vi "Create Group.vi"(4 "Channel Resources (Unset)":string[](array[string]), 5 "Raw Values (F)":bool, 6 "Channel Names":string[](array[string]), 7 "Group Type":refnum<class "Group.lvclass">, 8 "error in (no error)":errorcluster, 9 "Multicast Config (None)":T1, 10 "Group Info":T2, 11 "VolatusAPI in":refnum<class "VolatusAPI.lvclass">) -> (0 "error out":errorcluster, 2 "Group":refnum<class "Group.lvclass">, 3 "VolatusAPI out":refnum<class "VolatusAPI.lvclass">)   [LabVIEW 2020, in "Volatus.lvlib" / "VolatusAPI.lvclass"]
uses:
  VolatusAPI.lvclass
  lv-vecto/Vecto/Group Info.ctl
  lv-vecto/Vecto/Publish Config.ctl
  lv-vecto/Vecto/Group/Group.lvclass
  VolatusAPI.lvclass/VolatusAPI.ctl
  lv-vecto/Vecto/Channel Init.ctl
  lv-vecto/Vecto/ChannelService/Create Group Abstract.vi
  lv-vecto/Vecto/ChannelService/ChannelService.lvclass
  lv-vecto/Vecto/RemoteDataService/RemoteDataService.lvclass
  lv-vecto/VectoConfig/VectoConfig.lvlib
  lv-vecto/Vecto/Group Config/Group Config.lvclass
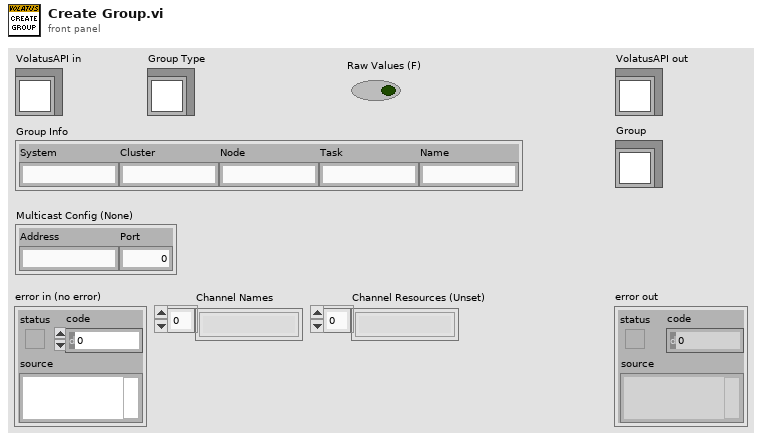
[diagram p1: front panel]
types:
  T1 = typedef "VectoConfig.lvlib/Publish Config.ctl" = cluster{"Address":string, "Port":u16}
  T2 = typedef "VectoConfig.lvlib/Group Info.ctl" = cluster{"System":string, "Cluster":string, "Node":string, "Task":string, "Name":string}
  T3 = typedef "VectoConfig.lvlib/Channel Init.ctl" = cluster{"Name":string, "Resource":string, "Unit String":string}
  T4 = typedef "VectoConfig.lvlib/Group Data Type.ctl" = enum16{"Double", "String", "Bool"}
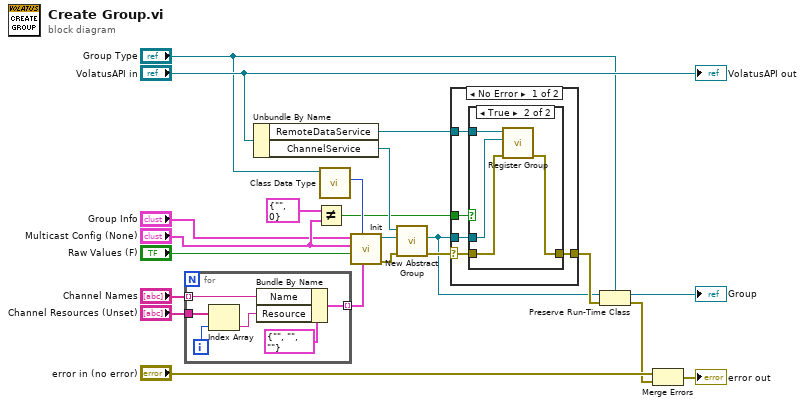
[diagram p0: block diagram]
diagram:
  n1 = for {
    tunnel: "Channel Names" -> [w24] mode=indexing
    tunnel: "Channel Resources (Unset)" -> [w27]
    tunnel: [w23] -> w20 mode=indexing
    i -> [w26]
    n2 = Index Array(array=w27, index=w26) -> (element=w25:string)
    n3 = Bundle By Name(cluster=T3 {"Name"="", "Resource"="", "Unit String"=""} ("Channel Init"), "Name"=w24, "Resource"=w25) -> (w23:T3)
  }
  n4 = Unbundle By Name("VolatusAPI in") -> ("RemoteDataService"=w4:refnum<class "RemoteDataService.lvclass">, "ChannelService"=w15:refnum<class "ChannelService.lvclass">)
  n5 = Not Equal?(x=T1 {"Address"="", "Port"=0}, y="Multicast Config (None)") -> (x != y?=w8:bool)
  n6 = call "Class Data Type.vi"("Group in"="Group Type") -> ("Class Data Type"=w14:T4)  [unwired: 8 in, 2 out]
  n7 = call "Init.vi"("Channels"=w20, "Group Data Type"=w14, "Raw Values (T)"="Raw Values (F)", "Multicast Endpoint (None)"="Multicast Config (None)", "Group Info"="Group Info") -> ("error out"=w17:errorcluster, "Group Config out"=w19:refnum<class "Group Config.lvclass">)  [unwired: 5 in]
  n8 = call "New Abstract Group.vi"("error in (no error)"=w17, "Group Config"=w19, "ChannelService in"=w15) -> ("error out"=w7:errorcluster, "Group"=w6:refnum<class "Group.lvclass">)  [unwired: 6 in, 1 out]
  n9 = case shown="No Error" w7 {
    selector: w7 -> [w30 w39]
    tunnel: w6 -> [w31 _]
    tunnel: w4 -> [w32 _]
    tunnel: w8 -> [w33 _]
    tunnel: [w29 w39] -> w22
    frame No Error {
      n10 = case shown="True" w33 {
        tunnel: w32 -> [_ w38]
        tunnel: w31 -> [_ w37]
        tunnel: w30 -> [w34 w36]
        tunnel: [w34 w35] -> w29
        frame False {
        }
        frame True {
          n11 = call "Register Group.vi"("error in (no error)"=w36, "Group"=w37, "RemoteDataService in"=w38) -> ("error out"=w35:errorcluster)  [unwired: 7 in, 1 out]
        }
      }
    }
    frame Error {
    }
  }
  n12 = Preserve Run-Time Class(object in=w6, error in=w22, 2:"Group Type") -> (object out=→"Group":refnum<class "Group.lvclass">, error out=w1:errorcluster)
  n13 = Merge Errors("error in (no error)", w1) -> (→"error out":errorcluster)
  "VolatusAPI out" <- "VolatusAPI in"
